vi "Register gRPC Methods.vi"(8 "error in (no error)":errorcluster, 11 "ServiceName Template in":refnum<class "ServiceName Template.lvclass">) -> (0 "error out":errorcluster, 3 "ServiceName Template out":refnum<class "ServiceName Template.lvclass">)   [LabVIEW 2024, in "ServiceName Template.lvclass"]
uses:
  ServiceName Template.lvclass
  ServiceName Template.lvclass/ServiceName Template.ctl
  typeDefs/Server Internal UEs.ctl
  typeDefs/Server gRPC UEs.ctl
  gRPC lv Support/grpc-lvsupport/grpcId.ctl
  gRPC lv Support/grpc-lvsupport/grpc-lvsupport.lvlib
  gRPC lv Support/grpc-lvsupport/gRPCId Cluster.ctl
  typeDefs/Server Internal Message.ctl
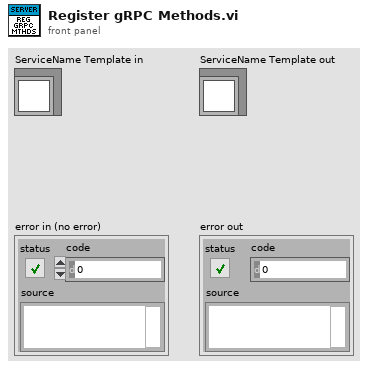
[diagram p1: front panel]
types:
  T1 = typedef "ServiceName Template.lvclass/Server gRPC UEs.ctl" = cluster{"package_service_method":refnum<user-event>}
  T2 = typedef "ServiceName Template.lvclass/Server Internal UEs.ctl" = cluster{"package_service_method Internal UE":refnum<user-event>}
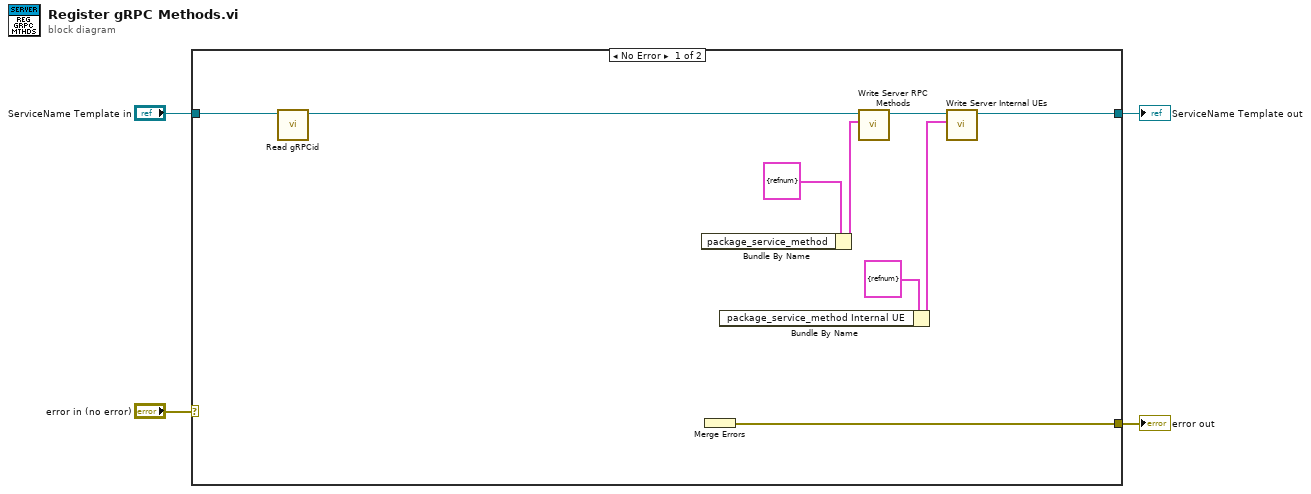
[diagram p0: block diagram]
diagram:
  n1 = case shown="No Error" "error in (no error)" {
    selector: "error in (no error)" -> [_ w14]
    tunnel: "ServiceName Template in" -> [w5 w15]
    tunnel: [w13 w14] -> w3
    tunnel: [w12 w15] -> w2
    frame No Error {
      n2 = call-dynamic "Read gRPCid.vi"("ServiceBase in"=w5) -> ("ServiceBase out"=w6:refnum<class "ServiceName Template.lvclass">)  [unwired: 8 in, 2 out]
      n3 = Bundle By Name ("Bundle gRPC UEs")(cluster=T1 {"package_service_method"=refnum} ("gRPC Server Method Events")) -> (w8:T1)  [unwired: 1 in]
      n4 = Merge Errors() -> (w13:errorcluster)  [unwired: 1 in]
      n5 = Bundle By Name ("Bundle Internal UEs")(cluster=T2 {"package_service_method Internal UE"=refnum} ("Server Internal UEs")) -> (w11:T2)  [unwired: 1 in]
      n6 = call "Write Server RPC Methods.vi"("Server RPC Methods"=w8, "ServiceName Template in"=w6) -> ("ServiceName Template out"=w9:refnum<class "ServiceName Template.lvclass">)  [unwired: 8 in, 1 out]
      n7 = call "Write Server Internal UEs.vi"("Server Internal UEs"=w11, "ServiceName Template in"=w9) -> ("ServiceName Template out"=w12:refnum<class "ServiceName Template.lvclass">)  [unwired: 8 in, 1 out]
    }
    frame Error {
    }
  }
  "error out" <- w3
  "ServiceName Template out" <- w2
